vi "Sub Initialize.vi"(8 "error in (no error)":errorcluster, 11 "Instrument Recorder in":refnum<class "Instrument Actor.lvclass">) -> (0 "error out":errorcluster, 2 "Initialize Result":refnum<class "Acquired Result.lvclass">, 3 "Instrument Recorder out":refnum<class "Instrument Actor.lvclass">)   [LabVIEW 2019, in "Instrument Actor.lvclass"]
uses:
  Instrument Actor.lvclass
  C:/GitHub/LabActor/Template Module/Template Module.lvclass
  C:/GitHub/LabActor/Worker/Worker.lvclass
  NHMFL_Core/Libraries/Instruments/Results/Acquired Result/Acquired Result.lvclass
  Instrument Actor.lvclass/Instrument Actor.ctl
  Template Module/Template Module.lvclass/Template Module.ctl
  Worker/Worker.lvclass/Worker.ctl
  NHMFL_Core/Libraries/Instruments/Instrument Driver/Instrument Driver.lvclass/Instrument Driver.ctl
  Read Instrument driver.vi
  Template Module/Read Configuration.vi
  Template Module/Read Name.vi
  Worker/Read Cycle period.vi
  NHMFL_Core/Libraries/Instruments/Instrument Driver/Write Recorder name.vi
  NHMFL_Core/Libraries/Instruments/Instrument Driver/Write Cycle period.vi
  Write Instrument driver.vi
  NHMFL_Core/Libraries/Instruments/Instrument Driver/Write User configuration.vi
  NHMFL_Core/Libraries/Instruments/Instrument Driver/Instrument Driver.lvclass
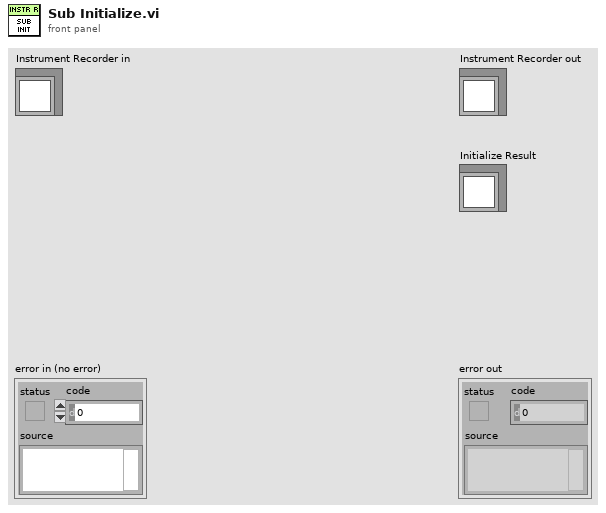
[diagram p1: front panel]
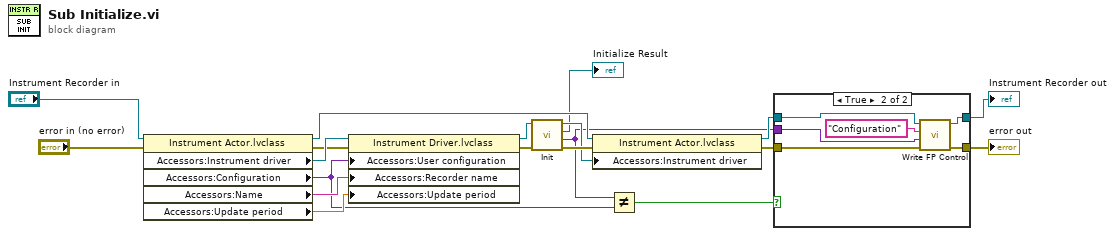
[diagram p0: block diagram]
diagram:
  n1 = property class="Instrument Actor.lvclass"(reference="Instrument Recorder in", error in="error in (no error)") -> (reference out=w18:refnum<class "Instrument Actor.lvclass">, error out=w11:errorcluster, "Accessors:Instrument driver"=w13:refnum<class "Instrument Driver.lvclass">, "Accessors:Configuration"=w2:variant, "Accessors:Name"=w9:string, "Accessors:Update period"=w8:dbl)
  n2 = property class="Instrument Driver.lvclass"(reference=w13, error in=w11, "Accessors:User configuration"=w2, "Accessors:Recorder name"=w9, "Accessors:Update period"=w8) -> (reference out=w12:refnum<class "Instrument Driver.lvclass">, error out=w10:errorcluster)
  n3 = call-dynamic "Init.vi"("error in (no error)"=w10, "Instrument Driver in"=w12) -> ("error out"=w16:errorcluster, "Post init configuration"=w3:variant, "Init Result"=→"Initialize Result":refnum<class "Acquired Result.lvclass">, "Instrument Driver out"=w15:refnum<class "Instrument Driver.lvclass">)  [unwired: 6 in]
  n4 = property class="Instrument Actor.lvclass"(reference=w18, error in=w16, "Accessors:Instrument driver"=w15) -> (reference out=w7:refnum<class "Instrument Actor.lvclass">, error out=w6:errorcluster)
  n5 = Not Equal?(x=w3, y=w2) -> (x != y?=w1:bool)
  n6 = case shown="True" w1 {
    tunnel: w7 -> [w21 w27]
    tunnel: w6 -> [w20 w26]
    tunnel: [w20 w25] -> w5
    tunnel: [w21 w24] -> w4
    tunnel: w3 -> [_ w22]
    frame False {
    }
    frame True {
      n7 = call-dynamic "Write FP Control.vi"("error in (no error)"=w26, "Control Value"=w22, "Control Name"="Configuration", "Measure Object in"=w27) -> ("error out"=w25:errorcluster, "Measure Object out"=w24:refnum<class "Instrument Actor.lvclass">)  [unwired: 6 in]
    }
  }
  "error out" <- w5
  "Instrument Recorder out" <- w4
